vi "ERP-ServerAddress.vi"() -> ()   [LabVIEW 2013]
panel:
  in  "Server Address":string
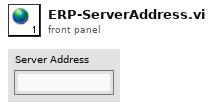
[diagram p1: front panel]
diagram:
